vi "Programmatically Reanimate.vi"() -> ()   [LabVIEW 2017]
doc: "A demonstration of programmatically reanimating a corpse (legacy code) to create a zombie at a grave (Diagram Disable Structure) using the Eulogy Toolkit API. The corpse is reanimated in the block diagram for the Reanimate - Simple.vi example."
uses:
  Toolkit VIs/Toolkit.lvlib
panel:
  in  "Stop Button":bool
  # "Overview: Demonstrates programmatically reanimating a grave using the Reanimate - Simple.vi as a target\nInstructions:\n1. Run the VI\n2. The Reanimate - Simple.vi's block diagram will be displayed\n3. The Corpse (legacy) frame of the grave will be reanimated (enabled) and the Spirit (refactored) frame will be disabled.\n4. Click the Stop button\n5. The programmatic reanimation will be undone to leave the Reanimate - Simple.vi example in its original state."
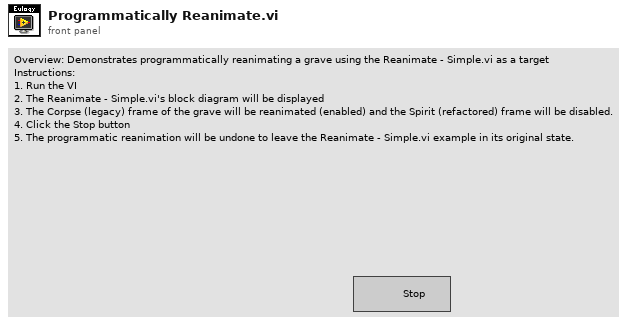
[diagram p1: front panel]
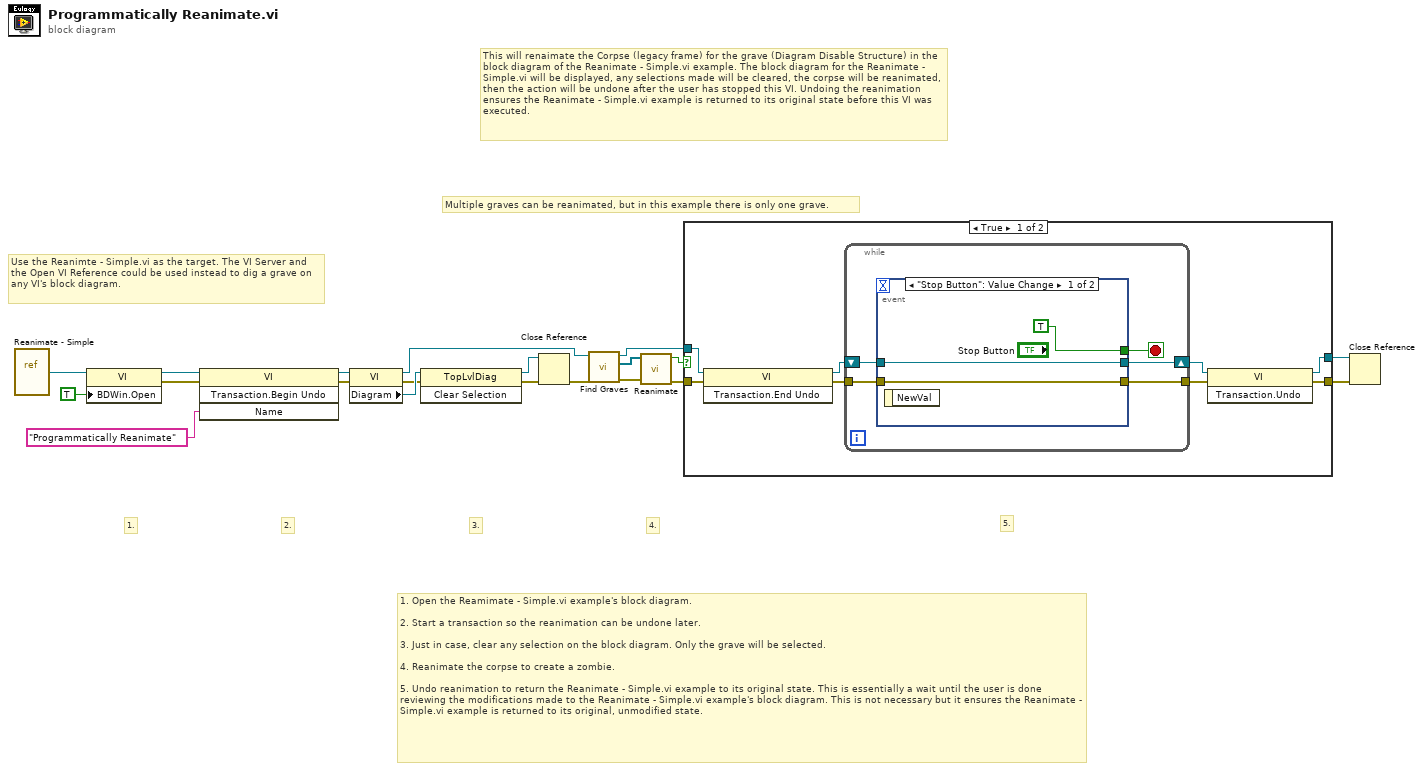
[diagram p0: block diagram]
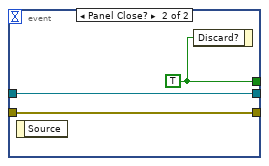
[diagram p2: hidden frame]
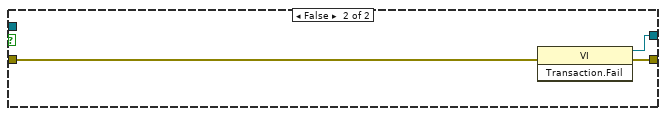
[diagram p3: hidden frame]
diagram:
  # "Multiple graves can be reanimated, but in this example there is only one grave."
  # "This will renaimate the Corpse (legacy frame) for the grave (Diagram Disable Structure) in the block diagram of the Reanimate - Simple.vi example. The block diagram for the Reanimate - Simple.vi will be displayed, any selections made will be cleared, the corpse will be reanimated, then the action will be undone after the user has stopped this VI. Undoing the reanimation ensures the Reanimate - Simple.vi example is returned to its original state before this VI was executed."
  # "Use the Reanimte - Simple.vi as the target. The VI Server and the Open VI Reference could be used instead to dig a grave on any VI's block diagram."
  # "1. Open the Reamimate - Simple.vi example's block diagram.\n\n2. Start a transaction so the reanimation can be undone later.\n\n3. Just in case, clear any selection on the block diagram. Only the grave will be selected.\n\n4. Reanimate the corpse to create a zombie.\n\n5. Undo reanimation to return the Reanimate - Simple.vi example to its original state. This is essentially a wait until the user is done reviewing the modifications made to the Reanimate - Simple.vi example's block diagram. This is not necessary but it ensures the Reanimate - Simple.vi example is returned to its original, unmodified state."
  # "5."
  # "4."
  # "3."
  # "2."
  # "1."
  n1 = vi-ref "Reanimate - Simple.vi"() -> (w17:refnum<vi>)
  n2 = property class="VI"(reference=w17, "BDWin.Open"=TRUE ("Block Diagram Window:Open")) -> (reference out=w16:refnum<vi>, error out=w14:errorcluster)  [unwired: 1 in]
  n3 = invoke class="VI" method="Transaction.Begin Undo"(reference=w16, error in=w14, "Name"="Programmatically Reanimate") -> (reference out=w13:refnum<vi>, error out=w12:errorcluster)  [unwired: 1 in, 2 out]
  n4 = property class="VI"(reference=w13, error in=w12) -> (reference out=w4:refnum<vi>, error out=w10:errorcluster, "Diagram"=w11:refnum<vi>)
  n5 = invoke class="TopLvlDiag" method="Clear Selection"(reference=w11, error in=w10) -> (reference out=w8:refnum<vi>, error out=w9:errorcluster)  [unwired: 1 in, 1 out]
  n6 = Close Reference(reference=w8, error in (no error)=w9) -> (error out=w5:errorcluster)
  n7 = call "Find Graves.vi"("Error In"=w5, "VI In"=w4) -> ("Error Out"=w1:errorcluster, "Graves"=w2:refnum<vi>[], "VI Out"=w3:refnum<vi>)  [unwired: 7 in]
  n8 = call "Reanimate.vi"("Error In"=w1, "Graves"=w2) -> ("Error Out"=w7:errorcluster, "Change Made?"=w6:bool)  [unwired: 8 in]
  n9 = case shown="True" w6 {
    tunnel: [w25 w42] -> w19
    tunnel: [w26 w41] -> w18
    tunnel: w3 -> [w22 _]
    tunnel: w7 -> [w21 w40]
    frame True {
      n10 = invoke class="VI" method="Transaction.End Undo"(reference=w22, error in=w21) -> (reference out=w28:refnum<vi>, error out=w24:errorcluster)  [unwired: 1 in, 1 out]
      n11 = while {
        shift-right: [w32] -> w27
        shift-left: w28 -> [w33]
        tunnel: w24 -> [w31]
        tunnel: [w30] -> w23
        stop <- w29 stop-if-true
        n12 = event shown="[0] \"Stop Button\": Value Change" {
          selector: _ -> [_ _]
          dyn-events: _ -> [_ _]
          timeout: _ -> [_ _]
          tunnel: w33 -> [w36 w39]
          tunnel: [w36 w39] -> w32
          tunnel: w31 -> [w35 w38]
          tunnel: [w35 w38] -> w30
          tunnel: [TRUE w37] -> w29
          event "Stop Button": Value Change {
            n13 = event-data() -> ()  [unwired: 1 in, 1 out]
          }
          event Panel Close? {
            w37 = TRUE
            n14 = event-data() -> ()  [unwired: 1 in, 1 out]
            n15 = event-data("Discard?"=w37) -> ()  [unwired: 1 in, 1 out]
          }
        }
      }
      n16 = invoke class="VI" method="Transaction.Undo"(reference=w27, error in=w23) -> (reference out=w26:refnum<vi>, error out=w25:errorcluster)  [unwired: 1 in, 1 out]
    }
    frame False {
      n17 = invoke class="VI" method="Transaction.Fail"(error in=w40) -> (reference out=w41:refnum<vi>, error out=w42:errorcluster)  [unwired: 2 in, 1 out]
    }
  }
  n18 = Close Reference(reference=w18, error in (no error)=w19) -> ()  [unwired: 1 out]
